vi "Scan lvclass.vi"(8 "error in (no error)":errorcluster, 10 "App Refnum":refnum<vi>, 11 "Path":path) -> (0 "error out":errorcluster, 1 "Accessors":string[](array[string]), 2 "Foreground Color":u32(colorbox), 3 "Public Events":string[](array[string]))   [LabVIEW 2016, in "LV Object Event Registration Node.xnode"]
uses:
  LV Object Event Registration Node.xnode
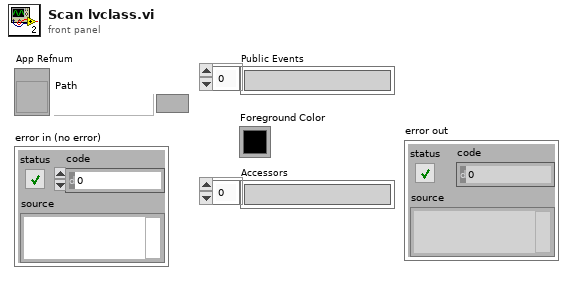
[diagram p1: front panel]
types:
  T1 = cluster{"Foreground Color":u32, "Background Color":u32, "Fill Pattern":cluster{"Row 0":u8, "Row 1":u8, "Row 2":u8, "Row 3":u8, "Row 4":u8, "Row 5":u8, "Row 6":u8, "Row 7":u8}, "Width":i16, "Mode":enum16{"Copy", "Or", "Exclusive Or", "Bit Clear", "Not Copy", "Not Or", "Nor Exclusive Or", "Not Bit Clear"}, "Style":enum32{"Solid", "Dash", "Dot", "Dash Dot", "Dash Dot Dot"}, "Fill Rule":enum32{"Even Odd", "Winding"}, "End Caps":enum32{"Default", "Flat"}}[]
  T2 = cluster{"Foreground Color":u32, "Background Color":u32, "Fill Pattern":cluster{"Row 0":u8, "Row 1":u8, "Row 2":u8, "Row 3":u8, "Row 4":u8, "Row 5":u8, "Row 6":u8, "Row 7":u8}, "Width":i16, "Mode":enum16{"Copy", "Or", "Exclusive Or", "Bit Clear", "Not Copy", "Not Or", "Nor Exclusive Or", "Not Bit Clear"}, "Style":enum32{"Solid", "Dash", "Dot", "Dash Dot", "Dash Dot Dot"}, "Fill Rule":enum32{"Even Odd", "Winding"}, "End Caps":enum32{"Default", "Flat"}}
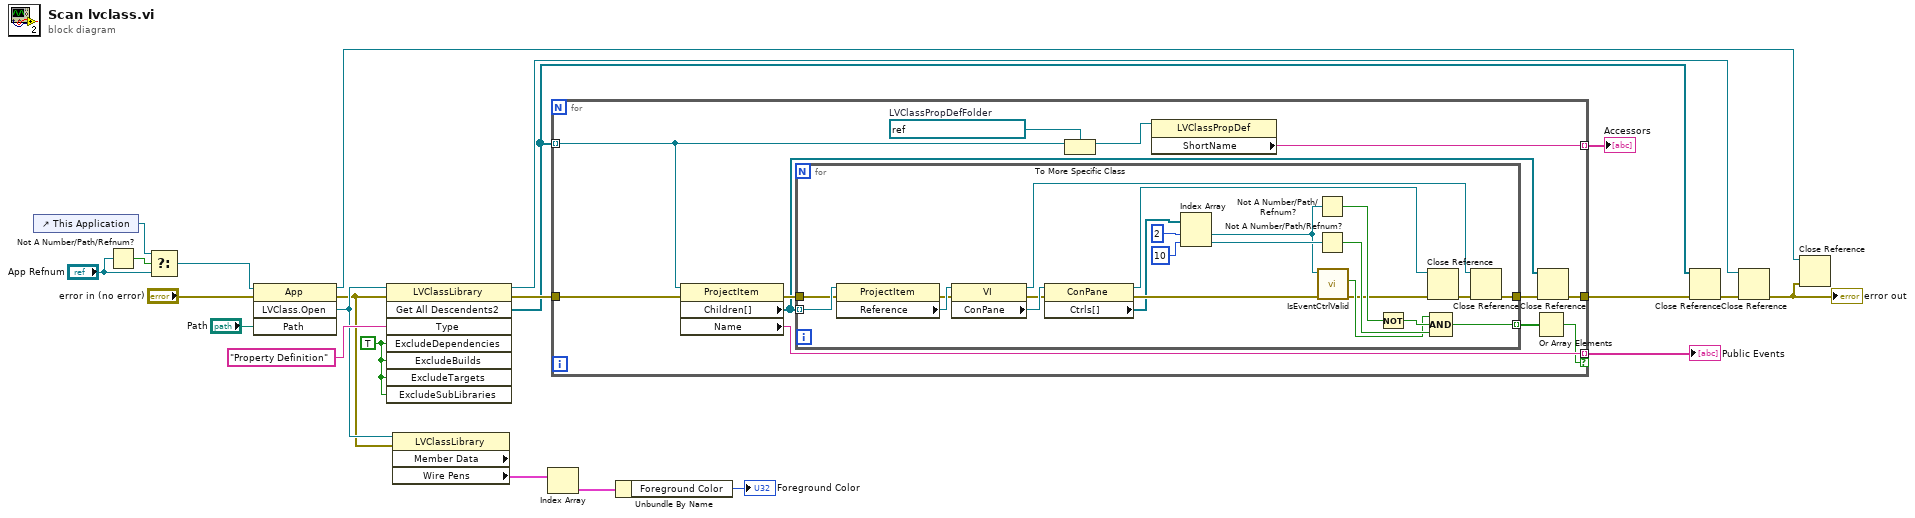
[diagram p0: block diagram]
diagram:
  w17 = TRUE ("ExcludeDependencies")
  n1 = control-ref of="This Application"() -> (w11:refnum<vi>)
  n2 = Not A Number/Path/Refnum?(number/path/refnum="App Refnum") -> (NaN/Path/Refnum?=w13:bool)
  n3 = Select(t=w11, s=w13, f="App Refnum") -> (s? t:f=w10:refnum<vi>)
  n4 = invoke class="App" method="LVClass.Open"(reference=w10, error in="error in (no error)", "Path"="Path") -> (reference out=w1:refnum<vi>, error out=w8:errorcluster, "LVClass.Open"=w15:refnum<vi>)  [unwired: 1 in, 1 out]
  n5 = invoke class="LVClassLibrary" method="Get All Descendents2"(reference=w15, error in=w8, "Type"="Property Definition", "ExcludeDependencies"=w17, "ExcludeBuilds"=w17, "ExcludeTargets"=w17, "ExcludeSubLibraries"=w17) -> (reference out=w4:refnum<vi>, error out=w7:errorcluster, "Get All Descendents2"=w6:refnum<vi>[])  [unwired: 1 in, 5 out]
  n6 = property class="LVClassLibrary" props=["Member Data", "Wire Pens"](reference=w15, error in=w8) -> ("Wire Pens"=w19:T1)  [unwired: 3 out]
  n7 = Index Array(array=w19) -> (element=w20:T2)  [unwired: 1 in]
  n8 = for {
    tunnel: w6 -> [w31] mode=indexing
    tunnel: [w32] -> w18 mode=indexing
    tunnel: [w29] -> w22 mode=indexing if=w28
    tunnel: w7 -> [w27]
    tunnel: [w23] -> w5
    w34 = refnum<vi> refnum  # LVClassPropDefFolder
    n9 = property class="ProjectItem"(reference=w31, error in=w27) -> (error out=w26:errorcluster, "Children[]"=w25:refnum<vi>[], "Name"=w29:string)  [unwired: 1 out]
    n10 = for {
      tunnel: w25 -> [w56] mode=indexing
      tunnel: [w46] -> w30 mode=indexing
      tunnel: [w35] -> w24
      tunnel: w26 -> [w43]
      n11 = property class="ProjectItem"(reference=w56, error in=w43) -> (error out=w42:errorcluster, "Reference"=w54:refnum<vi>)  [unwired: 1 out]
      n12 = property class="VI"(reference=w54, error in=w42) -> (reference out=w36:refnum<vi>, error out=w41:errorcluster, "ConPane"=w55:refnum<vi>)
      n13 = property class="ConPane"(reference=w55, error in=w41) -> (reference out=w38:refnum<vi>, error out=w47:errorcluster, "Ctrls[]"=w39:refnum<vi>[])
      n14 = Index Array(array=w39, index #1=2 ("index"), index #2=10 ("index")) -> (element #1=w44:refnum<vi>, element #2=w51:refnum<vi>)
      n15 = Not A Number/Path/Refnum?(number/path/refnum=w44) -> (NaN/Path/Refnum?=w50:bool)
      n16 = Not A Number/Path/Refnum?(number/path/refnum=w51) -> (NaN/Path/Refnum?=w48:bool)
      n17 = call "IsEventCtrlValid.vi"("error in (no error)"=w47, "Control in"=w44) -> ("error out"=w40:errorcluster, "Boolean"=w45:bool)  [unwired: 8 in]
      n18 = Not(x=w50) -> (.not. x?=w49:bool)
      n19 = Close Reference(reference=w38, error in (no error)=w40) -> (error out=w37:errorcluster)
      n20 = Compound Arithmetic op=AND(w45, w49, w48) -> (w46:bool)
      n21 = Close Reference(reference=w36, error in (no error)=w37) -> (error out=w35:errorcluster)
    }
    n22 = To More Specific Class(target class=w34, reference=w31) -> (specific class reference=w33:refnum<vi>)  [unwired: 1 in, 1 out]
    n23 = property class="LVClassPropDef"(reference=w33) -> ("ShortName"=w32:string)  [unwired: 1 in, 2 out]
    n24 = Or Array Elements(Boolean array=w30) -> (logical OR=w28:bool)
    n25 = Close Reference(reference=w25, error in (no error)=w24) -> (error out=w23:errorcluster)
  }
  "Public Events" <- w22
  "Accessors" <- w18
  n26 = Unbundle By Name(w20) -> ("Foreground Color"=→"Foreground Color":u32)
  n27 = Close Reference(reference=w6, error in (no error)=w5) -> (error out=w3:errorcluster)
  n28 = Close Reference(reference=w4, error in (no error)=w3) -> (error out=w2:errorcluster)
  "error out" <- w2
  n29 = Close Reference(reference=w1, error in (no error)=w2) -> ()  [unwired: 1 out]
